vi "Save Config.vi"(8 "error in":errorcluster, 11 "SignalConfig":T1={"VPP"=0, "Frecuency"=50.0, "Offset"=0.0, "signal type"=enum."Sine Wave"}) -> (0 "error out":errorcluster)   [LabVIEW 2020, in "DataBase.lvlib"]
uses:
  DataBase.lvlib
  Acquisition/SignalConfig--cluster.ctl
  <vilib>/drjdpowell/SQLite Library/SQL Connection/Open (path).vi
  <vilib>/drjdpowell/SQLite Library/SQL Connection/Open (string).vi
  <vilib>/AdvancedString/Path To Command Line String.vi
  <vilib>/drjdpowell/SQLite Library/SQL Connection/Execute SQL (No results).vi
  <vilib>/drjdpowell/SQLite Library/SQL Connection/Connection.lvclass
  <vilib>/drjdpowell/SQLite Library/SQLite.lvlib
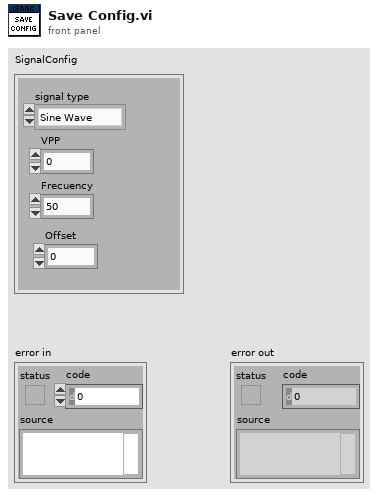
[diagram p1: front panel]
types:
  T1 = typedef "SignalConfig--cluster.ctl" = cluster{"VPP":i32, "Frecuency":dbl, "Offset":dbl, "signal type":enum16{"Sine Wave", "Triangle Wave", "Square Wave", "Sawtooth Wave"}}
  T2 = enum16{"Sine Wave", "Triangle Wave", "Square Wave", "Sawtooth Wave"}
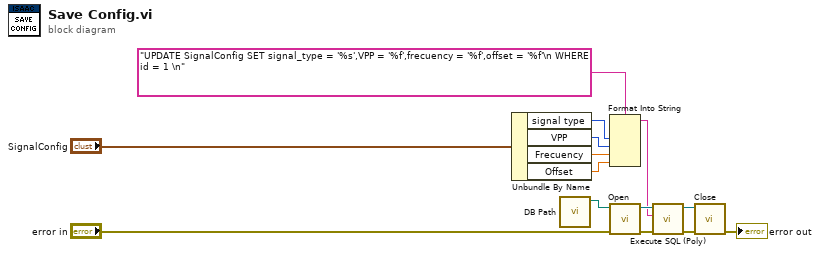
[diagram p0: block diagram]
diagram:
  n1 = Unbundle By Name("SignalConfig") -> ("signal type"=w5:T2, "VPP"=w4:i32, "Frecuency"=w3:dbl, "Offset"=w2:dbl)
  n2 = call "DB Path.vi"() -> ("appended path"=w6:path)  [unwired: 11 in]
  n3 = Format Into String(format string="UPDATE SignalConfig SET signal_type = '%s',VPP = '%f',frecuency = '%f',offset = '%f'\n WHERE id = 1 \n", w5, w4, w3, w2) -> (resulting string=w8:string)  [unwired: 2 in, 1 out]
  n4 = call-poly <vilib>:"Open.vi"("error in (no error)"="error in", "db file"=w6) -> ("error out"=w14:errorcluster, "SQLite Connection"=w10:refnum<class "Connection.lvclass">)  [unwired: 8 in]
  n5 = call-poly <vilib>:"Execute SQL (Poly).vi"("error in (no error)"=w14, "SQL"=w8, "SQLite Connection in"=w10) -> ("error out"=w13:errorcluster, "SQLite Connection"=w9:refnum<class "Connection.lvclass">)  [unwired: 7 in]
  n6 = call-dynamic "Close.vi"("error in (no error)"=w13, "SQLite Connection in"=w9) -> ("error out"=→"error out":errorcluster)  [unwired: 9 in]
